vi "Init Gmail OAuth2.vi"(5 "Scopes (gmail.send)":string[](array[string])=["https://www.googleapis.com/auth/gmail.send"], 7 "Redirect URL (http://localhost)":string, 10 "Client":refnum<class "Client.lvclass">, 11 "Account (Prompt)":string) -> (3 "OAuth2 out":refnum<class "OAuth2.lvclass">)   [LabVIEW 2020, in "Gmail API.lvlib" / "OAuth2.lvclass"]
uses:
  OAuth2.lvclass
  C:/Program Files (x86)/National Instruments/LabVIEW 2020/vi.lib/IlluminatedG/IG HTTP Utils/OAuth2/OAuth2/OAuth2.lvclass
  <vilib>/IlluminatedG/IG HTTP Utils/OAuth2/Client/Client.lvclass
  <vilib>/IlluminatedG/IG HTTP Utils/OAuth2/Request/Request.lvclass
  <vilib>/IlluminatedG/IG HTTP Utils/OAuth2/OAuth2/OAuth2.lvclass
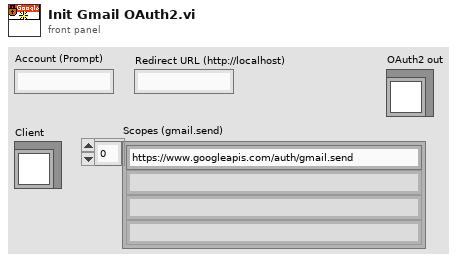
[diagram p1: front panel]
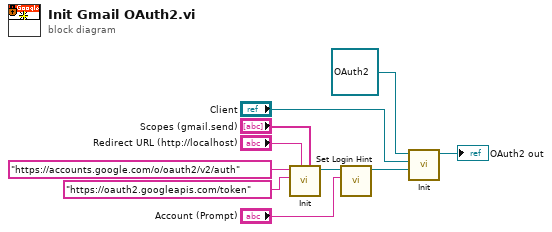
[diagram p0: block diagram]
diagram:
  n1 = call <vilib>:"Init.vi"("Scopes"="Scopes (gmail.send)", "Redirect URL (http://localhost)"="Redirect URL (http://localhost)", "Token URL"="https://oauth2.googleapis.com/token" ("url"), "Auth URL"="https://accounts.google.com/o/oauth2/v2/auth" ("url")) -> ("Request out"=w6:refnum<class "Request.lvclass">)  [unwired: 7 in]
  n2 = call <vilib>:"Set Login Hint.vi"("Login Hint"="Account (Prompt)", "Request in"=w6) -> ("Request out"=w4:refnum<class "Request.lvclass">)  [unwired: 9 in]
  n3 = call <vilib>:"Init.vi"("Request"=w4, "Client"="Client", "OAuth2 in (New)"=refnum<class "OAuth2.lvclass"> refnum ("OAuth2 in")) -> ("OAuth2"=→"OAuth2 out":refnum<class "OAuth2.lvclass">)  [unwired: 8 in]
